vi "Check LOG flag.vi"(8 "error in (no error)":errorcluster, 10 "status message":string, 11 "ICS in":refnum<class "ICS.lvclass">) -> (0 "error out":errorcluster, 2 "LOG status":bool, 3 "ICS out":refnum<class "ICS.lvclass">)   [LabVIEW 2018, in "ICS.lvclass"]
uses:
  ICS.lvclass
  ICS.lvclass/ICS.ctl
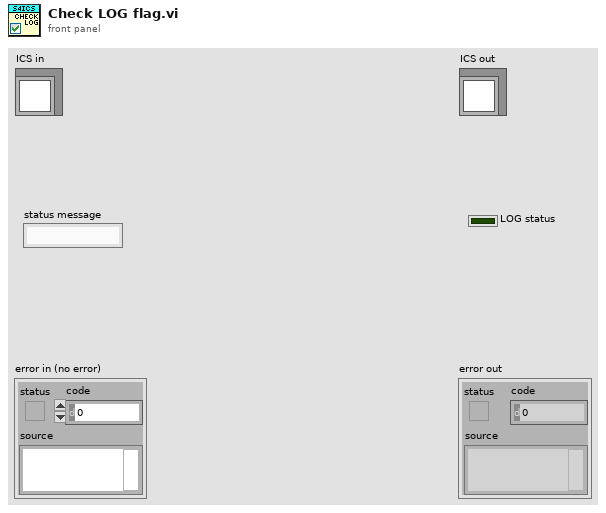
[diagram p1: front panel]
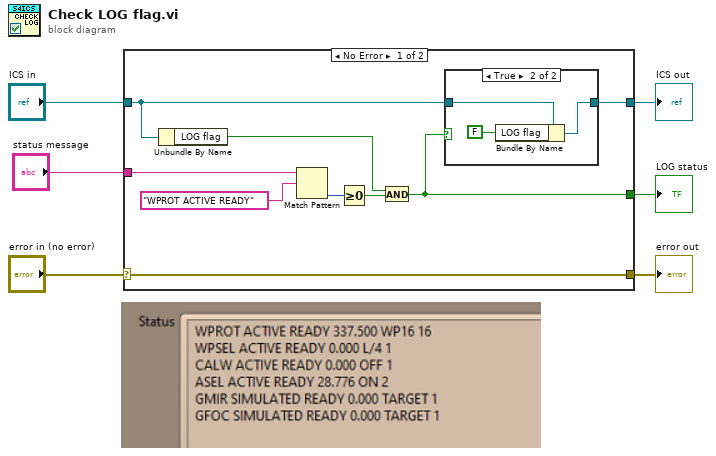
[diagram p0: block diagram]
diagram:
  n1 = case shown="No Error" "error in (no error)" {
    selector: "error in (no error)" -> [w15 w20]
    tunnel: [w15 w20] -> w5
    tunnel: [w7 w21] -> w3
    tunnel: "ICS in" -> [w8 w21]
    tunnel: "status message" -> [w13 _]
    tunnel: [w9 _] -> w1
    frame No Error {
      n2 = Unbundle By Name(w8) -> ("LOG flag"=w10:bool)
      n3 = Match Pattern(string=w13, regular expression="WPROT ACTIVE READY") -> (offset past match=w14:i32)  [unwired: 1 in, 3 out]
      n4 = Greater Or Equal To 0?(x=w14) -> (x >= 0?=w11:bool)
      n5 = And(x=w10, y=w11) -> (x .and. y?=w9:bool)
      n6 = case shown="True" w9 {
        tunnel: w8 -> [w16 w19]
        tunnel: [w16 w18] -> w7
        frame False {
        }
        frame True {
          n7 = Bundle By Name(cluster=w19, "LOG flag"=FALSE) -> (w18:refnum<class "ICS.lvclass">)
        }
      }
    }
    frame Error {
    }
  }
  "error out" <- w5
  "ICS out" <- w3
  "LOG status" <- w1
